vi "Get Project Items New.vi"(8 "error in (no error)":errorcluster, 11 "Path":path) -> (0 "error out":errorcluster, 3 "Items Data":refnum<class "Item.lvclass">[](array[class]))   [LabVIEW 2020, in "VI Properties Editor.lvlib"]
uses:
  VI Properties Editor.lvlib
  Classes/Item/Item.lvclass
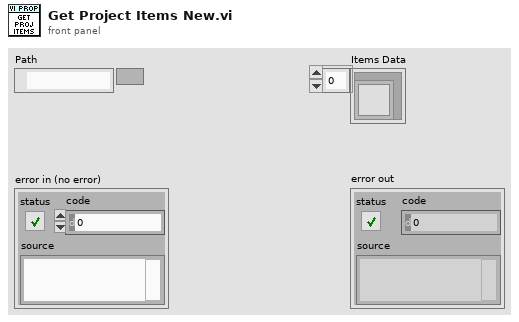
[diagram p1: front panel]
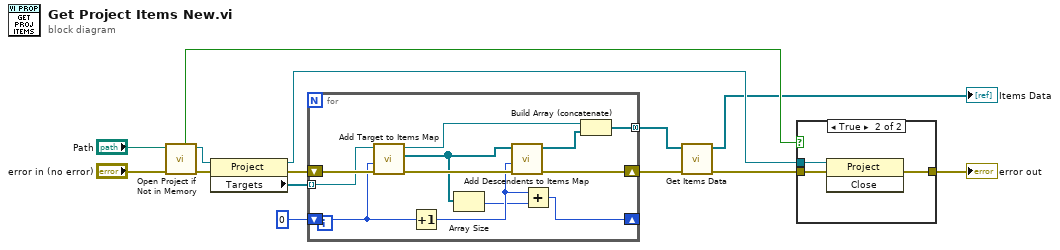
[diagram p0: block diagram]
diagram:
  n1 = call "Open Project if Not in Memory.vi"("error in (no error)"="error in (no error)", "Path"="Path") -> ("error out"=w10:errorcluster, "Project Ref"=w8:refnum<vi>, "Opened?"=w5:bool)  [unwired: 7 in]
  n2 = property class="Project"(reference=w8, error in=w10) -> (reference out=w11:refnum<vi>, error out=w14:errorcluster, "Targets"=w13:refnum<vi>[])
  n3 = for {
    tunnel: w13 -> [w18] mode=indexing
    shift-right: [w24] -> w12
    shift-left: w14 -> [w26]
    shift-right: [w20] -> _
    shift-left: 0 -> [w23]
    tunnel: [w15] -> w1 mode=concatenating
    n4 = call "Add Target to Items Map.vi"("error in (no error)"=w26, "Order"=w23, "TargetItem Ref"=w18) -> ("error out"=w25:errorcluster, "Descendents Refs"=w19:refnum<vi>[], "Item"=w17:refnum<class "Item.lvclass">)  [unwired: 6 in]
    n5 = Increment(x=w23) -> (x+1=w22:i32)
    n6 = Array Size(array=w19) -> (size(s)=w21:i32)
    n7 = call "Add Descendents to Items Map.vi"("error in (no error)"=w25, "Order"=w22, "Descendents Refs"=w19) -> ("error out"=w24:errorcluster, "Items"=w16:refnum<class "Item.lvclass">[])  [unwired: 7 in]
    n8 = Add(x=w22, y=w21) -> (x+y=w20:i32)
    n9 = Build Array (concatenate)(w17, w16) -> (w15:refnum<class "Item.lvclass">[])
  }
  n10 = call "Get Items Data.vi"("error in (no error)"=w12, "Items"=w1) -> ("error out"=w4:errorcluster, "Items out"=→"Items Data":refnum<class "Item.lvclass">[])  [unwired: 8 in]
  n11 = case shown="True" w5 {
    tunnel: w4 -> [w27 w30]
    tunnel: w11 -> [_ w29]
    tunnel: [w27 w28] -> w6
    frame False {
    }
    frame True {
      n12 = invoke class="Project" method="Close"(reference=w29, error in=w30) -> (error out=w28:errorcluster)  [unwired: 1 in, 2 out]
    }
  }
  "error out" <- w6
